vi "Verify if an automatic New Page just appends.vi"(0 "PDF Report IN":refnum<class "PDF Report Class.lvclass">, 11 "error in (no error)":errorcluster) -> (4 "PDF Report OUT":refnum<class "PDF Report Class.lvclass">, 15 "error out":errorcluster)   [LabVIEW 2019]
doc: "Version 1.0\nDeveloped by Jean-Marc Simard\nCopyright © 2010, Exaprom Inc.\nAll rights reserved.\nLicense: BSD\n\nWith iTextSharp 4.1.6 (http://itextsharp.sourceforge.net)\nunder Mozilla Public License Version 1.1\n(http://www.mozilla.org/MPL/MPL-1.1.html)"
uses:
  <userlib>/Exaprom PDF/LV Class/PDF Report Class/PDF Report Class.lvclass
  C:/Program Files/National Instruments/LabVIEW 2019/user.lib/Exaprom PDF/DLL/itextsharp.dll
  DLL/itextsharp.dll
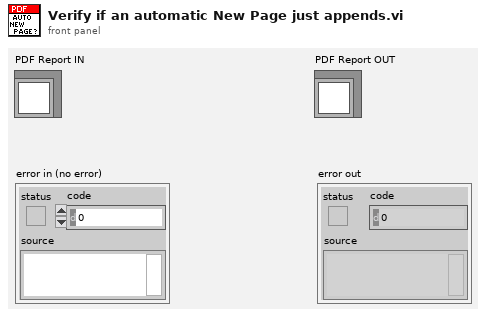
[diagram p1: front panel]
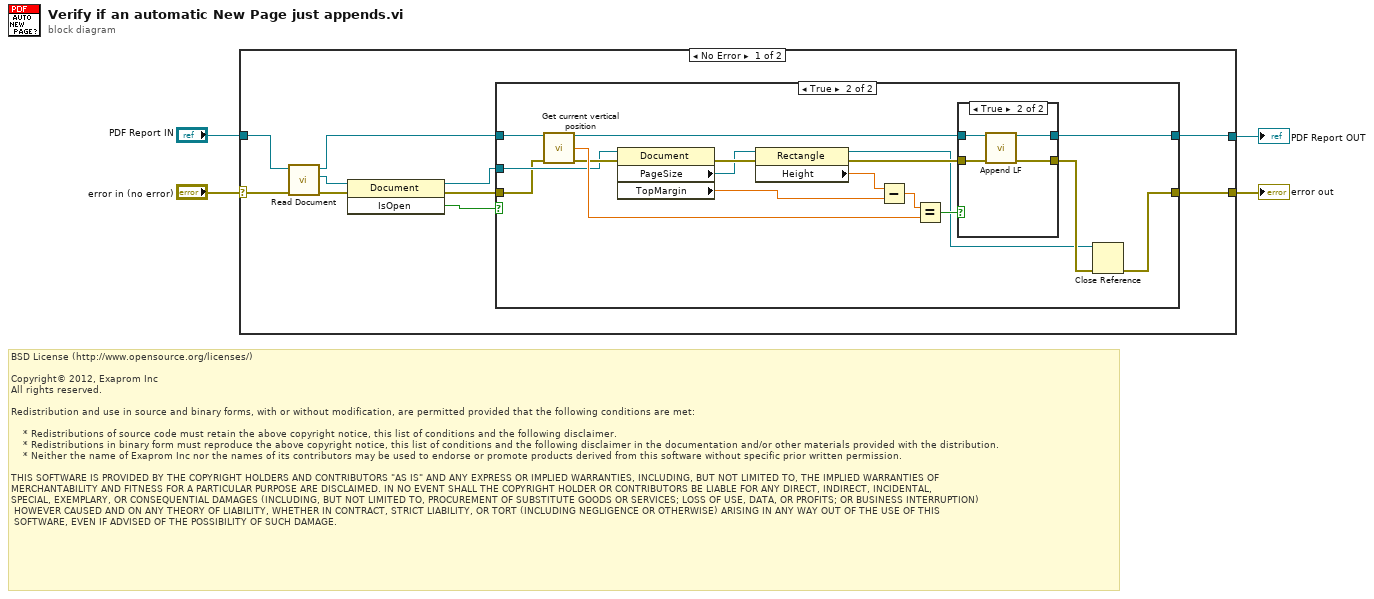
[diagram p0: block diagram]
diagram:
  # "BSD License (http://www.opensource.org/licenses/)\n\nCopyright© 2012, Exaprom Inc\nAll rights reserved.\n\nRedistribution and use in source and binary forms, with or without modification, are permitted provided that the following conditions are met:\n\n    * Redistributions of source code must retain the above copyright notice, this list of conditions and the following disclaimer.\n    * Redistributions in binary form must reproduce the above copyright notice, this list of conditions and the following disclaimer in the documentation and/or other materials provided with the distribution.\n    * Neither the name of Exaprom Inc nor the names of its contributors may be used to endorse or promote products derived from this software without specific prior written permission.\n\nTHIS SOFTWARE IS PROVIDED BY THE COPYRIGHT HOLDERS AND CONTRIBUTORS \"AS IS\" AND ANY EXPRESS OR IMPLIED WARRANTIES, INCLUDING, BUT NOT LIMITED TO, THE IMPLIED WARRANTIES OF \nMERCHANTABILITY AND FITNESS FOR A PARTICULAR PURPOSE ARE DISCLAIMED. IN NO EVENT SHALL THE COPYRIGHT HOLDER OR CONTRIBUTORS BE LIABLE FOR ANY DIRECT, INDIRECT, INCIDENTAL,\nSPECIAL, EXEMPLARY, OR CONSEQUENTIAL DAMAGES (INCLUDING, BUT NOT LIMITED TO, PROCUREMENT OF SUBSTITUTE GOODS OR SERVICES; LOSS OF USE, DATA, OR PROFITS; OR BUSINESS INTERRUPTION)\n HOWEVER CAUSED AND ON ANY THEORY OF LIABILITY, WHETHER IN CONTRACT, STRICT LIABILITY, OR TORT (INCLUDING NEGLIGENCE OR OTHERWISE) ARISING IN ANY WAY OUT OF THE USE OF THIS\n SOFTWARE, EVEN IF ADVISED OF THE POSSIBILITY OF SUCH DAMAGE."
  n1 = case shown="No Error" "error in (no error)" {
    selector: "error in (no error)" -> [w10 w41]
    tunnel: "PDF Report IN" -> [w8 w40]
    tunnel: [w14 w40] -> w3
    tunnel: [w13 w41] -> w2
    frame No Error {
      n2 = call-dynamic "Read Document.vi"("error in (no error)"=w10, "PDF Report Class in"=w8) -> ("error out"=w9:errorcluster, "Document"=w7:refnum<k24>, "PDF Report Class out"=w6:refnum<class "PDF Report Class.lvclass">)  [unwired: 7 in]
      n3 = invoke class="Document" method="IsOpen"(reference=w7, error in=w9) -> (reference out=w5:refnum<k24>, error out=w11:errorcluster, "IsOpen"=w12:bool)  [unwired: 1 in]
      n4 = case shown="True" w12 {
        tunnel: w6 -> [w16 w33]
        tunnel: [w16 w26] -> w14
        tunnel: [w15 w19] -> w13
        tunnel: w5 -> [_ w21]
        tunnel: w11 -> [w15 w20]
        frame False {
        }
        frame True {
          n5 = call <userlib>:"Get current vertical position.vi"("PDF Report In"=w33, "error in (no error)"=w20) -> ("PDF Report duplicate"=w27:refnum<class "PDF Report Class.lvclass">, "GetVerticalPosition (points)"=w29:sgl, "error out"=w25:errorcluster)  [unwired: 1 in, 10 out]
          n6 = property class="Document"(reference=w21, error in=w25) -> (error out=w24:errorcluster, "PageSize"=w17:refnum<k24>, "TopMargin"=w31:sgl)  [unwired: 1 out]
          n7 = property class="Rectangle"(reference=w17, error in=w24) -> (reference out=w18:refnum<k24>, error out=w23:errorcluster, "Height"=w32:sgl)
          n8 = Subtract(x=w32, y=w31) -> (x-y=w30:sgl)
          n9 = Equal?(x=w30, y=w29) -> (x = y?=w28:bool)
          n10 = case shown="True" w28 {
            tunnel: w27 -> [w35 w39]
            tunnel: [w35 w38] -> w26
            tunnel: w23 -> [w34 w37]
            tunnel: [w34 w36] -> w22
            frame False {
            }
            frame True {
              n11 = call <userlib>:"Append LF.vi"("PDF Report IN"=w39, "error in (no error)"=w37) -> ("PDF Report duplicate"=w38:refnum<class "PDF Report Class.lvclass">, "error out"=w36:errorcluster)  [unwired: 2 in, 10 out]
            }
          }
          n12 = Close Reference(reference=w18, error in (no error)=w22) -> (error out=w19:errorcluster)
        }
      }
    }
    frame Error {
    }
  }
  "PDF Report OUT" <- w3
  "error out" <- w2
